vi "Setup subWorker - DAQ Worker.vi"(8 "error in":errorcluster, 11 "ChartView in":refnum<class "ChartView.lvclass">) -> (0 "error out":errorcluster, 3 "ChartView out":refnum<class "ChartView.lvclass">)   [LabVIEW 2020, in "ChartView.lvclass"]
doc: "This VI sets up the framework parameters of a statically-linked subWorker."
uses:
  ChartView.lvclass
  ChartView.lvclass/ChartView.ctl
  DAQ Worker/DAQ Worker.lvclass
  C:/Program Files (x86)/National Instruments/LabVIEW 2020/vi.lib/addons/_Workers/Library/Classes/Worker/Worker.lvclass
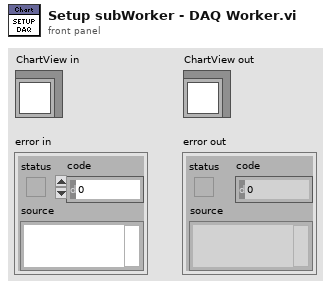
[diagram p1: front panel]
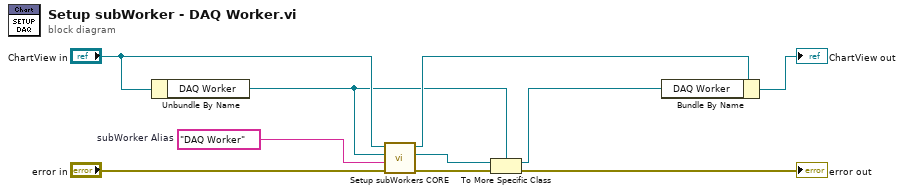
[diagram p0: block diagram]
diagram:
  w6 = "DAQ Worker"  # subWorker Alias
  n1 = Unbundle By Name("ChartView in") -> ("DAQ Worker"=w3:refnum<class "DAQ Worker.lvclass">)
  n2 = call-dynamic "Setup subWorkers CORE.vi"("error in"="error in", "subWorker Alias"=w6, "subWorker"=w3, "Worker"="ChartView in") -> ("error out"=w5:errorcluster, "subWorker out"=w1:refnum<class "Worker.lvclass">, "Worker out"=w8:refnum<class "ChartView.lvclass">)  [unwired: 5 in]
  n3 = To More Specific Class(target class=w3, reference=w1, error in=w5) -> (specific class reference=w2:refnum<class "DAQ Worker.lvclass">, error out=→"error out":errorcluster)
  n4 = Bundle By Name(cluster=w8, "DAQ Worker"=w2) -> (→"ChartView out":refnum<class "ChartView.lvclass">)
